vi "ROI_point2corner.vi"(11 "appended array":dbl[](array[numeric])) -> (3 "Array":dbl[][](array[numeric]))   [LabVIEW 2017]
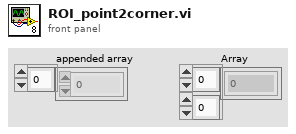
[diagram p1: front panel]
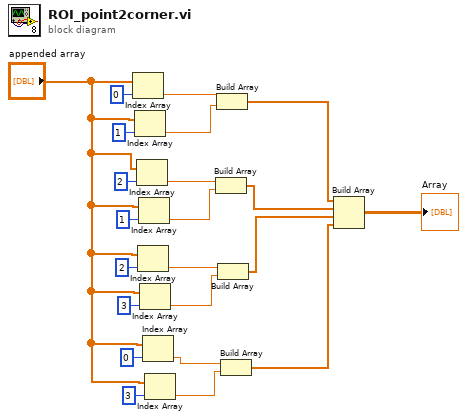
[diagram p0: block diagram]
diagram:
  n1 = Index Array(array="appended array", index=0) -> (element=w9:dbl)
  n2 = Index Array(array="appended array", index=1) -> (element=w11:dbl)
  n3 = Index Array(array="appended array", index=2) -> (element=w12:dbl)
  n4 = Index Array(array="appended array", index=2) -> (element=w14:dbl)
  n5 = Index Array(array="appended array", index=1) -> (element=w13:dbl)
  n6 = Index Array(array="appended array", index=3) -> (element=w15:dbl)
  n7 = Index Array(array="appended array", index=0) -> (element=w16:dbl)
  n8 = Index Array(array="appended array", index=3) -> (element=w17:dbl)
  n9 = Build Array(w12, w13) -> (w19:dbl[])
  n10 = Build Array(w9, w11) -> (w18:dbl[])
  n11 = Build Array(w14, w15) -> (w20:dbl[])
  n12 = Build Array(w16, w17) -> (w21:dbl[])
  n13 = Build Array(w18, w19, w20, w21) -> (→"Array":dbl[][])
